vi "Autonomous Independent.vi"   [LabVIEW 2017]
doc: "This VI is called when autonomous begins, and will automatically be terminated when autonomous ends. You can carry out timed or sensor driven robot movement independently without needing to return to the caller."
uses:
  <vilib>/Rock Robotics/Network Tables/NT Read String.vi
  <vilib>/Rock Robotics/WPI/Utilities/WPI_GetSetVariantRefNum.vi
  <vilib>/Rock Robotics/Network Tables/NT Read Number.vi
  Robot Global Data.vi
panel:
  # "Be sure to right-click and choose Data Operations>>Make Current Value default if you want to save the array values with the VI"
types:
  T1 = typedef "WPI_RobotDriveDevRef.ctl" = cluster{"DevStatus":errorcluster, "Motors[]":T2[], "Square Inputs":bool, "Max Output":dbl}
  T2 = typedef "WPI_MotorControlDeviceRef.ctl" = cluster{"DeviceStatus":errorcluster, "Type":T3, "PWM":cluster{"PWM Channel":T4, "DeadBand":T5}, "CAN":cluster{"Device Number":u8, "SetOutput VI Ref":variant, "GetOutput VI Ref":variant, "Enable VI Ref":variant, "Disable VI Ref":variant, "Data":variant}, "Invert":bool, "DIO PWM":cluster{"PWM \"Enable\" Channel":T4, "DIOChannel":T6, "PWM Rate":dbl}}
  T3 = typedef "WPI_MotorControlType.ctl" = enum16{"PWM", "CAN", "DIO PWM"}
  T4 = typedef "FPGA_DIOPWMChannel.ctl" = enum8{"PWM 0", "PWM 1", "PWM 2", "PWM 3", "PWM 4", "PWM 5", "PWM 6", "PWM 7", "PWM 8", "PWM 9", "PWM MXP 0", "PWM MXP 1", "PWM MXP 2", "PWM MXP 3", "PWM MXP 4", "PWM MXP 5", "PWM MXP 6", "PWM MXP 7", "PWM MXP 8", "PWM MXP 9", "Invalid"}
  T5 = typedef "WPI_PWMDeadband.ctl" = cluster{"Name":string, "maxPositivePwm":i32, "minPositivePwm":i32, "centerPwm":i32, "maxNegativePwm":i32, "minNegativePwm":i32, "angularRange":u16}
  T6 = typedef "FPGA_DIOChannel.ctl" = enum8{"DIO 0", "DIO 1", "DIO 2", "DIO 3", "DIO 4", "DIO 5", "DIO 6", "DIO 7", "DIO 8", "DIO 9", "DIO MXP 0", "DIO MXP 1", "DIO MXP 2", "DIO MXP 3", "DIO MXP 4", "DIO MXP 5", "DIO MXP 6", "DIO MXP 7", "DIO MXP 8", "DIO MXP 9", "DIO MXP 10", "DIO MXP 11", "DIO MXP 12", "DIO MXP 13", "DIO MXP 14", "DIO MXP 15", "SPI Port CS1", "SPI Port CS2", "SPI Port CS3", "SPI Port MISO", "SPI Port MOSI", "Invalid"}
  T7 = typedef "WPI_DigitalInputDevRef.ctl" = cluster{"DevStatus":errorcluster, "DIO Channel":T6}
  T8 = typedef "WPI_GyroDevRef.ctl" = cluster{"DevStatus":errorcluster, "Analog Channel":T9, "Gain (VoltsPerDegree/Second)":dbl, "Gyro Type":enum16{"Analog", "XRS450"}, "Handle":i32, "SPI Bus":T10, "Device Found":bool, "Sample Rate":dbl, "Calibrate On Open":bool, "Offset":dbl}
  T9 = typedef "FPGA_AIChannel.ctl" = enum8{"AI 0", "AI 1", "AI 2", "AI 3", "AI MXP 0", "AI MXP 1", "AI MXP 2", "AI MXP 3", "Invalid"}
  T10 = typedef "spi_bus.ctl" = enum16{"SPI On-Board, CS0", "SPI On-Board, CS1", "SPI On-Board, CS2", "SPI On-Board, CS3", "SPI MXP", "Invalid"}
  T11 = typedef "WPI_EncoderDevRef.ctl" = cluster{"DevStatus":errorcluster, "EncoderIndex":T12, "CounterIndex":T13, "DistancePerCount":dbl, "Decoding Type":T14}
  T12 = typedef "FPGA_EncoderIdx.ctl" = enum8{"Enc 0", "Enc 1", "Enc 2", "Enc 3", "Enc 4", "Enc 5", "Enc 6", "Enc 7", "Invalid"}
  T13 = typedef "FPGA_CounterCtrSystemIndex.ctl" = enum8{"Ctr 0", "Ctr 1", "Ctr 2", "Ctr 3", "Ctr 4", "Ctr 5", "Ctr 6", "Ctr 7", "Invalid"}
  T14 = typedef "WPI_EncoderType.ctl" = enum16{"1x", "2x", "4x"}
  T15 = cluster{"Axes[0]":dbl, "Axes[1]":dbl, "Axes[2]":dbl, "Axes[3]":dbl, "Axes[4]":dbl, "Axes[5]":dbl, "Axes[6]":dbl, "Axes[7]":dbl, "Axes[8]":dbl}
  T16 = cluster{"CHECKSUM":u16, "SIGNATURE NUMBER":u16, "X CENTER":u16, "Y CENTER":u16, "TRAGET WIDTH":u16, "TARGET HEIGHT":u16, "X_LOCK":bool, "Y_LOCK":bool}
diagram:
  (unwired) "This function is run in parallel when the autonomous period begins. It will be terminated automatically when the period ends.\n\nNote that all Driver Station inputs are automatically latched and will not change once auto begins."
  # "This tells you the autonomous selected\nfrom the dashboard"
  # "Every 20ms, report that we are running autonomous\ncode. Loop will abort the same time as the VI."
  # "Use time and/or sensors to control how the robot drives."
  # "This tells you the driver position\nand alliance color"
  n1 = while {
    tunnel: [w29] -> w9
    tunnel: [w30] -> w6
    i -> [w25]
    stop <- w20 stop-if-true
    n2 = call <vilib>:"WPI_DriverStationGame Specific Data.vi"() -> ("Game Specific Data"=w35:string)  [unwired: 11 in]
    n3 = call <vilib>:"WPI_DriverStationGame Specific Data.vi"() -> ("Game Specific Data"=w33:string)  [unwired: 11 in]
    n4 = Wait (ms)(milliseconds to wait=u32 10) -> ()  [unwired: 1 out]
    n5 = String Subset(string=w35, length (rest)=1 ("length (rest)")) -> (substring=w29:string)  [unwired: 1 in]
    n6 = String Subset(string=w33, offset (0)=1, length (rest)=1 ("length (rest)")) -> (substring=w30:string)
    n7 = String Length(string=w29) -> (length=w27:i32)
    n8 = String Length(string=w30) -> (length=w28:i32)
    n9 = Greater Than 0?(x=w27) -> (x > 0?=w23:bool)
    n10 = Greater Than 0?(x=w28) -> (x > 0?=w22:bool)
    n11 = Greater Or Equal?(x=w25, y=500) -> (x >= y?=w21:bool)
    n12 = Compound Arithmetic op=OR(w23, w22, w21) -> (w20:bool)
  }
  n13 = call <vilib>:"WPI_DriverStationGet Alliance Info.vi"() -> ()  [unwired: 12 out]
  n14 = while {
    stop <- FALSE stop-if-true
    n15 = call <vilib>:"WPI_DriverStationReport Robot Code State.vi"("Autonomous"=TRUE) -> ()  [unwired: 10 in, 1 out]
    n16 = Wait (ms)(milliseconds to wait=u32 20) -> ()  [unwired: 1 out]
  }
  n17 = global write "Robot Global Data.vi" "Current State"(TRUE ("Current State")) -> ()
  n18 = call <vilib>:"WPI_RobotDriveRefNum Registry Get.vi"("refnum name"="Left and Right Motors") -> ("RobotDriveDevRef"=w12:T1)  [unwired: 9 in, 1 out]
  n19 = call-poly <vilib>:"NT Read Value.vi"("Name"="DB/Slider 0" ("refnum name")) -> ("Numeric"=w7:dbl)  [unwired: 9 in, 1 out]
  n20 = call-poly <vilib>:"NT Read Value.vi"("Name"="DB/Slider 1" ("refnum name")) -> ("Numeric"=w4:dbl)  [unwired: 9 in, 1 out]
  n21 = call-poly <vilib>:"NT Read Value.vi"("Name"="Auto Selector") -> ("String"=w18:string)  [unwired: 9 in, 1 out]
  n22 = call <vilib>:"WPI_DigitalInputRefNum Registry Get.vi"("refnum name"="Infrared") -> ("DigitalInputDevRef"=w1:T7)  [unwired: 9 in, 1 out]
  n23 = call <vilib>:"WPI_GyroRefNum Registry Get.vi"("refnum name"="Gyro") -> ("GyroDevRef"=w10:T8)  [unwired: 9 in, 1 out]
  n24 = call <vilib>:"WPI_EncoderRefNum Registry Get.vi"("refnum name"="Left") -> ("EncoderDevRef"=w15:T11)  [unwired: 9 in, 1 out]
  n25 = call <vilib>:"WPI_EncoderRefNum Registry Get.vi"("refnum name"="Right") -> ("EncoderDevRef"=w14:T11)  [unwired: 9 in, 1 out]
  n26 = case shown="\"Right Scale V2\"" w18 {
    tunnel: w15 -> [w47 w86 w449 w1297 w1563 w1948 w2679 w3428 w4238 w4503 w4890 w5156 w5885 w6662 w7471 w7729 w7754 w7788 w7814]
    tunnel: w14 -> [w46 w87 w450 w1296 w1562 w1949 w2680 w3427 w4237 w4504 w4889 w5155 w5884 w6661 w7472 w7728 w7753 w7789 w7813]
    tunnel: w12 -> [w45 w88 w452 w1299 w1564 w1946 w2677 w3430 w4236 w4502 w4892 w5158 w5887 w6664 w7473 w7730 w7756 w7786 w7811]
    tunnel: w10 -> [w41 w85 w451 w1298 w1565 w1947 w2678 w3429 w4239 w4501 w4891 w5157 w5886 w6663 w7470 w7731 w7755 w7787 w7812]
    tunnel: w9 -> [_ w83 w453 w1293 w1559 w1951 w2675 w3424 w4235 w4499 w4886 w5153 w5890 w6658 w7469 _ _ _ _]
    tunnel: w7 -> [w39 w78 w448 w1295 w1561 w1945 w2676 w3426 w4234 w4505 w4888 w5159 w5888 w6660 w7464 w7725 w7750 w7790 w7816]
    tunnel: w6 -> [_ _ _ w1294 w1560 w1950 w2674 w3425 _ w4500 w4887 w5154 w5889 w6659 _ _ _ _ _]
    tunnel: w4 -> [_ _ _ _ _ _ _ _ _ _ _ _ _ _ _ _ w7749 _ w7810]
    tunnel: w1 -> [_ _ _ _ _ _ _ w3423 _ _ _ _ _ w6657 _ _ _ _ w7815]
    frame "Autoline", Default {
      n27 = flat-sequence {
        tunnel: w47 -> [w63]
        tunnel: w46 -> [w62]
        tunnel: w45 -> [w61]
        tunnel: [w60] -> w44
        tunnel: [w59] -> w43
        tunnel: [w58] -> w42
        tunnel: w41 -> [w57]
        tunnel: [w56] -> w40
        tunnel: w39 -> [w53]
        tunnel: w40 -> [w66]
        tunnel: w42 -> [w65]
        tunnel: w43 -> [w64]
        tunnel: w44 -> [w67]
        frame #0 {
          n28 = Multiply(x=w53, y=1000.0) -> (x*y=w50:dbl)
          n29 = Wait (ms)(milliseconds to wait=10) -> ()  [unwired: 1 out]
          n30 = call <vilib>:"WPI_EncoderReset.vi"("EncoderDevRef"=w62) -> ("EncoderDevRef"=w58:T11)  [unwired: 9 in, 1 out]
          n31 = Equal?(x=w50, y=0.0) -> (x = y?=w51:bool)
          n32 = Greater?(x=w50, y=11000.0) -> (0:w52:bool)
          n33 = call <vilib>:"WPI_RobotDriveTankDrive.vi"("RobotDriveDevRef"=w61) -> ("RobotDriveDevRef"=w60:T1)  [unwired: 8 in, 2 out]
          n34 = Or(x=w52, y=w51) -> ()  [unwired: 1 out]
          n35 = call <vilib>:"WPI_GyroReset.vi"("GyroDevRef"=w57) -> ("GyroDevRef"=w56:T8)  [unwired: 9 in, 1 out]
          n36 = call <vilib>:"WPI_EncoderReset.vi"("EncoderDevRef"=w63) -> ("EncoderDevRef"=w59:T11)  [unwired: 9 in, 1 out]
        }
        frame #1 {
          n37 = flat-sequence {
            tunnel: w67 -> [w73]
            tunnel: w66 -> [w72]
            tunnel: w65 -> [w70]
            tunnel: [w71] -> w68
            tunnel: w64 -> [w69]
            tunnel: w68 -> [w76]
            frame #0 {
              n38 = call "PID Distance.vi"("Distance"=90.0, "Angle"=0.0, "RightEncoder"=w69, "LeftEncoder"=w70, "GyroDevRef"=w72, "RobotDriveDevRef"=w73) -> ("RobotDriveDevRef 2"=w71:T1)  [unwired: 2 in, 3 out]
            }
            frame #1 {
              w77 = 0.0
              n39 = call <vilib>:"WPI_RobotDriveTankDrive.vi"("Right axis value"=w77, "Left axis value"=w77, "RobotDriveDevRef"=w76) -> ()  [unwired: 6 in, 3 out]
            }
          }
        }
      }
    }
    frame "Center Switch" {
      n40 = flat-sequence {
        tunnel: [w110] -> w84
        tunnel: [w109] -> w82
        tunnel: [w108] -> w81
        tunnel: [w107] -> w80
        tunnel: [w106] -> w79
        tunnel: w78 -> [w104]
        tunnel: w83 -> [w110]
        tunnel: w85 -> [w111]
        tunnel: w86 -> [w112]
        tunnel: w87 -> [w113]
        tunnel: w88 -> [w114]
        tunnel: w84 -> [w120]
        tunnel: w82 -> [w119]
        tunnel: w81 -> [w118]
        tunnel: w80 -> [w117]
        tunnel: w79 -> [w116]
        frame #0 {
          w115 = 0.0 ("Left axis value")
          # "Section 1:\nCode initialization"
          n41 = global read "Robot Global Data.vi" "Axes"() -> (w95:dbl[])
          n42 = call <vilib>:"WPI_RobotDriveTankDrive.vi"("Right axis value"=w115, "Left axis value"=w115, "RobotDriveDevRef"=w114) -> ("RobotDriveDevRef"=w109:T1)  [unwired: 6 in, 2 out]
          n43 = global write "Robot Global Data.vi" "Lift_Position"(0.0) -> ()
          n44 = Multiply(x=w104, y=1000.0) -> (x*y=w99:dbl)
          n45 = global write "Robot Global Data.vi" "Raise_Mast"(FALSE ("Current State")) -> ()
          n46 = global write "Robot Global Data.vi" "Current State"(TRUE ("Current State")) -> ()
          n47 = global write "Robot Global Data.vi" "Raise_Mast"(FALSE ("Current State")) -> ()
          n48 = Array To Cluster(array=w95) -> (cluster=w94:T15)
          n49 = Bundle By Name(cluster=w94, "Axes[1]"=-1.0) -> (w93:T15)
          n50 = Greater?(x=w99, y=11000.0) -> (0:w101:bool)
          n51 = Equal?(x=w99, y=0.0) -> (x = y?=w102:bool)
          n52 = Or(x=w101, y=w102) -> ()  [unwired: 1 out]
          n53 = Cluster To Array(cluster=w93) -> (array=w92:dbl[])
          n54 = call <vilib>:"WPI_GyroReset.vi"("GyroDevRef"=w111) -> ("GyroDevRef"=w108:T8)  [unwired: 9 in, 1 out]
          n55 = call <vilib>:"WPI_EncoderReset.vi"("EncoderDevRef"=w112) -> ("EncoderDevRef"=w106:T11)  [unwired: 9 in, 1 out]
          n56 = global write "Robot Global Data.vi" "Axes"(w92) -> ()
          n57 = call <vilib>:"WPI_EncoderReset.vi"("EncoderDevRef"=w113) -> ("EncoderDevRef"=w107:T11)  [unwired: 9 in, 1 out]
          n58 = Wait (ms)(milliseconds to wait=0) -> ()  [unwired: 1 out]
        }
        frame #1 {
          n59 = case shown="\"L\"" w120 {
            tunnel: w119 -> [w140 w281 w302]
            tunnel: w118 -> [w141 w280 w303]
            tunnel: w117 -> [w143 w278 w304]
            tunnel: w116 -> [w142 w279 w305]
            frame "R" {
              n60 = flat-sequence {
                tunnel: [w168] -> w164
                tunnel: [w167] -> w163
                tunnel: [w166] -> w162
                tunnel: [w165] -> w161
                tunnel: w143 -> [w169]
                tunnel: w142 -> [w170]
                tunnel: w141 -> [w172]
                tunnel: w140 -> [w171]
                tunnel: [w180] -> w160
                tunnel: w164 -> [w179]
                tunnel: [w178] -> w159
                tunnel: w163 -> [w178]
                tunnel: [w177] -> w158
                tunnel: w162 -> [w177]
                tunnel: [w176] -> w157
                tunnel: w161 -> [w176]
                tunnel: [w183] -> w139
                tunnel: [w184] -> w137
                tunnel: w160 -> [w185]
                tunnel: w159 -> [w186]
                tunnel: [w190] -> w135
                tunnel: w158 -> [w190]
                tunnel: [w189] -> w133
                tunnel: w157 -> [w189]
                tunnel: w139 -> [w199]
                tunnel: [w199] -> w138
                tunnel: w137 -> [w198]
                tunnel: [w193] -> w136
                tunnel: w135 -> [w197]
                tunnel: [w194] -> w134
                tunnel: w133 -> [w196]
                tunnel: [w195] -> w132
                tunnel: w138 -> [w207]
                tunnel: w136 -> [w206]
                tunnel: w134 -> [w204]
                tunnel: w132 -> [w205]
                tunnel: [w202] -> w156
                tunnel: [w203] -> w155
                tunnel: [w201] -> w154
                tunnel: [w200] -> w153
                tunnel: [w211] -> w152
                tunnel: [w212] -> w151
                tunnel: w156 -> [w220]
                tunnel: w155 -> [w219]
                tunnel: [w223] -> w150
                tunnel: w154 -> [w223]
                tunnel: [w222] -> w149
                tunnel: w153 -> [w222]
                tunnel: [w235] -> w148
                tunnel: [w234] -> w147
                tunnel: [w233] -> w146
                tunnel: w152 -> [w233]
                tunnel: [w232] -> w145
                tunnel: w151 -> [w232]
                tunnel: w150 -> [w225]
                tunnel: w149 -> [w224]
                tunnel: w148 -> [w240]
                tunnel: w147 -> [w239]
                tunnel: w146 -> [w242]
                tunnel: w145 -> [w241]
                tunnel: [w243] -> w144
                tunnel: [w238] -> w127
                tunnel: [w237] -> w124
                tunnel: [w236] -> w121
                tunnel: w144 -> [w257]
                tunnel: [w249] -> w130
                tunnel: [w248] -> w128
                tunnel: w127 -> [w248]
                tunnel: [w247] -> w125
                tunnel: w124 -> [w247]
                tunnel: [w246] -> w122
                tunnel: w121 -> [w246]
                tunnel: [w262] -> w131
                tunnel: w130 -> [w262]
                tunnel: [w261] -> w129
                tunnel: w128 -> [w261]
                tunnel: [w260] -> w126
                tunnel: w125 -> [w260]
                tunnel: [w259] -> w123
                tunnel: w122 -> [w259]
                tunnel: w123 -> [w268]
                tunnel: w126 -> [w267]
                tunnel: w129 -> [w266]
                tunnel: w131 -> [w265]
                frame #0 {
                  n61 = call "PID Distance.vi"("Distance"=20.0, "Angle"=0.0, "RightEncoder"=w169, "LeftEncoder"=w170, "GyroDevRef"=w172, "RobotDriveDevRef"=w171) -> ("RightEncoder 2"=w165:T11, "LeftEncoder 2"=w166:T11, "GyroDevRef 2"=w167:T8, "RobotDriveDevRef 2"=w168:T1)  [unwired: 2 in]
                }
                frame #1 {
                  w181 = 0.0 ("Left axis value")
                  n62 = global write "Robot Global Data.vi" "Raise_Mast"(TRUE ("Current State")) -> ()
                  n63 = Wait (ms)(milliseconds to wait=u32 100) -> ()  [unwired: 1 out]
                  n64 = call <vilib>:"WPI_RobotDriveTankDrive.vi"("Right axis value"=w181, "Left axis value"=w181, "RobotDriveDevRef"=w179) -> ("RobotDriveDevRef"=w180:T1)  [unwired: 6 in, 2 out]
                }
                frame #2 {
                  n65 = call "PID turning.vi"("Angle"=45.0, "GyroDevRef"=w186, "RobotDriveDevRef"=w185) -> ("GyroDevRef 2"=w183:T8, "RobotDriveDevRef 2"=w184:T1)  [unwired: 7 in]
                  n66 = global write "Robot Global Data.vi" "Raise_Mast"(TRUE ("Current State")) -> ()
                }
                frame #3 {
                  w192 = 0.0 ("Left axis value")
                  n67 = call <vilib>:"WPI_EncoderReset.vi"("EncoderDevRef"=w197) -> ("EncoderDevRef"=w194:T11)  [unwired: 9 in, 1 out]
                  n68 = call <vilib>:"WPI_EncoderReset.vi"("EncoderDevRef"=w196) -> ("EncoderDevRef"=w195:T11)  [unwired: 9 in, 1 out]
                  n69 = Wait (ms)(milliseconds to wait=u32 10) -> ()  [unwired: 1 out]
                  n70 = call <vilib>:"WPI_RobotDriveTankDrive.vi"("Right axis value"=w192, "Left axis value"=w192, "RobotDriveDevRef"=w198) -> ("RobotDriveDevRef"=w193:T1)  [unwired: 6 in, 2 out]
                }
                frame #4 {
                  n71 = call "PID Distance.vi"("Distance"=60.0, "Angle"=45.0, "RightEncoder"=w205, "LeftEncoder"=w204, "GyroDevRef"=w207, "RobotDriveDevRef"=w206) -> ("RightEncoder 2"=w200:T11, "LeftEncoder 2"=w201:T11, "GyroDevRef 2"=w203:T8, "RobotDriveDevRef 2"=w202:T1)  [unwired: 2 in]
                  n72 = global write "Robot Global Data.vi" "Raise_Mast"(TRUE ("Current State")) -> ()
                }
                frame #5 {
                  n73 = global read "Robot Global Data.vi" "Axes"() -> (w217:dbl[])
                  n74 = global write "Robot Global Data.vi" "Raise_Mast"(TRUE ("Current State")) -> ()
                  n75 = Array To Cluster(array=w217) -> (cluster=w218:T15)
                  n76 = Bundle By Name(cluster=w218, "Axes[1]"=-1.0) -> (w215:T15)
                  n77 = Cluster To Array(cluster=w215) -> (array=w216:dbl[])
                  n78 = call "PID turning.vi"("Angle"=0.0, "GyroDevRef"=w219, "RobotDriveDevRef"=w220) -> ("GyroDevRef 2"=w211:T8, "RobotDriveDevRef 2"=w212:T1)  [unwired: 7 in]
                  n79 = global write "Robot Global Data.vi" "Axes"(w216) -> ()
                }
                frame #6 {
                  n80 = global read "Robot Global Data.vi" "Axes"() -> (w227:dbl[])
                  n81 = global write "Robot Global Data.vi" "Lift_Position"(2.0) -> ()
                  n82 = Array To Cluster(array=w227) -> (cluster=w226:T15)
                  n83 = Bundle By Name(cluster=w226, "Axes[1]"=-1.0) -> (w229:T15)
                  n84 = Cluster To Array(cluster=w229) -> (array=w228:dbl[])
                  n85 = call <vilib>:"WPI_EncoderReset.vi"("EncoderDevRef"=w224) -> ("EncoderDevRef"=w234:T11)  [unwired: 9 in, 1 out]
                  n86 = global write "Robot Global Data.vi" "Axes"(w228) -> ()
                  n87 = call <vilib>:"WPI_EncoderReset.vi"("EncoderDevRef"=w225) -> ("EncoderDevRef"=w235:T11)  [unwired: 9 in, 1 out]
                }
                frame #7 {
                  n88 = call "PID Distance.vi"("Distance"=50.0, "Angle"=0.0, "RightEncoder"=w239, "LeftEncoder"=w240, "GyroDevRef"=w242, "RobotDriveDevRef"=w241) -> ("RightEncoder 2"=w236:T11, "LeftEncoder 2"=w237:T11, "GyroDevRef 2"=w238:T8, "RobotDriveDevRef 2"=w243:T1)  [unwired: 2 in]
                }
                frame #8 {
                  w258 = 0.0 ("Left axis value")
                  n89 = global read "Robot Global Data.vi" "Axes"() -> (w254:dbl[])
                  n90 = global write "Robot Global Data.vi" "Lift_Position"(2.0) -> ()
                  n91 = Wait (ms)(milliseconds to wait=u32 500) -> ()  [unwired: 1 out]
                  n92 = Array To Cluster(array=w254) -> (cluster=w253:T15)
                  n93 = Bundle By Name(cluster=w253, "Axes[1]"=1.0) -> (w251:T15)
                  n94 = Cluster To Array(cluster=w251) -> (array=w250:dbl[])
                  n95 = call <vilib>:"WPI_RobotDriveTankDrive.vi"("Right axis value"=w258, "Left axis value"=w258, "RobotDriveDevRef"=w257) -> ("RobotDriveDevRef"=w249:T1)  [unwired: 6 in, 2 out]
                  n96 = global write "Robot Global Data.vi" "Axes"(w250) -> ()
                }
                frame #9 {
                  n97 = global write "Robot Global Data.vi" "Current State"(FALSE ("Current State")) -> ()
                  n98 = Wait (ms)(milliseconds to wait=u32 500) -> ()  [unwired: 1 out]
                }
                frame #10 {
                  n99 = global read "Robot Global Data.vi" "Axes"() -> (w276:dbl[])
                  n100 = call "PID Distance.vi"("Distance"=20.0, "Angle"=0.0, "RightEncoder"=w268, "LeftEncoder"=w267, "GyroDevRef"=w266, "RobotDriveDevRef"=w265) -> ()  [unwired: 2 in, 4 out]
                  n101 = global write "Robot Global Data.vi" "Lift_Position"(0.0) -> ()
                  n102 = Array To Cluster(array=w276) -> (cluster=w275:T15)
                  n103 = Bundle By Name(cluster=w275, "Axes[1]"=-1.0) -> (w273:T15)
                  n104 = Cluster To Array(cluster=w273) -> (array=w272:dbl[])
                  n105 = global write "Robot Global Data.vi" "Axes"(w272) -> ()
                }
              }
            }
            frame Default {
              n106 = flat-sequence {
                tunnel: w281 -> [w286]
                tunnel: w280 -> [w285]
                tunnel: w279 -> [w283]
                tunnel: w278 -> [w282]
                tunnel: [w284] -> w277
                tunnel: w277 -> [w289]
                frame #0 {
                  n107 = call "PID Distance.vi"("Distance"=90.0, "Angle"=0.0, "RightEncoder"=w282, "LeftEncoder"=w283, "GyroDevRef"=w285, "RobotDriveDevRef"=w286) -> ("RobotDriveDevRef 2"=w284:T1)  [unwired: 2 in, 3 out]
                }
                frame #1 {
                  w290 = 0.0
                  n108 = call <vilib>:"WPI_RobotDriveTankDrive.vi"("Right axis value"=w290, "Left axis value"=w290, "RobotDriveDevRef"=w289) -> ()  [unwired: 6 in, 3 out]
                }
              }
            }
            frame "L" {
              n109 = flat-sequence {
                tunnel: [w338] -> w334
                tunnel: [w337] -> w333
                tunnel: [w336] -> w332
                tunnel: [w335] -> w331
                tunnel: w304 -> [w339]
                tunnel: w305 -> [w340]
                tunnel: w303 -> [w342]
                tunnel: w302 -> [w341]
                tunnel: [w350] -> w330
                tunnel: w334 -> [w349]
                tunnel: [w348] -> w329
                tunnel: w333 -> [w348]
                tunnel: [w347] -> w328
                tunnel: w332 -> [w347]
                tunnel: [w346] -> w327
                tunnel: w331 -> [w346]
                tunnel: [w354] -> w326
                tunnel: [w355] -> w325
                tunnel: w330 -> [w356]
                tunnel: w329 -> [w353]
                tunnel: [w360] -> w324
                tunnel: w328 -> [w360]
                tunnel: [w359] -> w323
                tunnel: w327 -> [w359]
                tunnel: w326 -> [w369]
                tunnel: [w369] -> w322
                tunnel: w325 -> [w368]
                tunnel: [w363] -> w321
                tunnel: w324 -> [w367]
                tunnel: [w364] -> w320
                tunnel: w323 -> [w366]
                tunnel: [w365] -> w319
                tunnel: w322 -> [w377]
                tunnel: w321 -> [w376]
                tunnel: w320 -> [w374]
                tunnel: w319 -> [w375]
                tunnel: [w372] -> w318
                tunnel: [w373] -> w317
                tunnel: [w371] -> w316
                tunnel: [w370] -> w315
                tunnel: [w381] -> w314
                tunnel: [w382] -> w313
                tunnel: w318 -> [w391]
                tunnel: w317 -> [w390]
                tunnel: [w394] -> w312
                tunnel: w316 -> [w394]
                tunnel: [w393] -> w311
                tunnel: w315 -> [w393]
                tunnel: [w406] -> w310
                tunnel: [w405] -> w309
                tunnel: [w404] -> w308
                tunnel: w314 -> [w404]
                tunnel: [w403] -> w307
                tunnel: w313 -> [w403]
                tunnel: w312 -> [w396]
                tunnel: w311 -> [w395]
                tunnel: w310 -> [w411]
                tunnel: w309 -> [w410]
                tunnel: w308 -> [w413]
                tunnel: w307 -> [w412]
                tunnel: [w414] -> w306
                tunnel: [w409] -> w297
                tunnel: [w408] -> w294
                tunnel: [w407] -> w291
                tunnel: w306 -> [w428]
                tunnel: [w420] -> w300
                tunnel: [w419] -> w298
                tunnel: w297 -> [w419]
                tunnel: [w418] -> w295
                tunnel: w294 -> [w418]
                tunnel: [w417] -> w292
                tunnel: w291 -> [w417]
                tunnel: [w433] -> w301
                tunnel: w300 -> [w433]
                tunnel: [w432] -> w299
                tunnel: w298 -> [w432]
                tunnel: [w431] -> w296
                tunnel: w295 -> [w431]
                tunnel: [w430] -> w293
                tunnel: w292 -> [w430]
                tunnel: w301 -> [w439]
                tunnel: w299 -> [w438]
                tunnel: w296 -> [w437]
                tunnel: w293 -> [w436]
                frame #0 {
                  n110 = call "PID Distance.vi"("Distance"=20.0, "Angle"=0.0, "RightEncoder"=w339, "LeftEncoder"=w340, "GyroDevRef"=w342, "RobotDriveDevRef"=w341) -> ("RightEncoder 2"=w335:T11, "LeftEncoder 2"=w336:T11, "GyroDevRef 2"=w337:T8, "RobotDriveDevRef 2"=w338:T1)  [unwired: 2 in]
                }
                frame #1 {
                  w351 = 0.0 ("Left axis value")
                  n111 = global write "Robot Global Data.vi" "Raise_Mast"(TRUE ("Current State")) -> ()
                  n112 = Wait (ms)(milliseconds to wait=u32 100) -> ()  [unwired: 1 out]
                  n113 = call <vilib>:"WPI_RobotDriveTankDrive.vi"("Right axis value"=w351, "Left axis value"=w351, "RobotDriveDevRef"=w349) -> ("RobotDriveDevRef"=w350:T1)  [unwired: 6 in, 2 out]
                }
                frame #2 {
                  n114 = call "PID turning.vi"("Angle"=-50.0, "GyroDevRef"=w353, "RobotDriveDevRef"=w356) -> ("GyroDevRef 2"=w354:T8, "RobotDriveDevRef 2"=w355:T1)  [unwired: 7 in]
                  n115 = global write "Robot Global Data.vi" "Raise_Mast"(TRUE ("Current State")) -> ()
                }
                frame #3 {
                  w362 = 0.0 ("Left axis value")
                  n116 = call <vilib>:"WPI_EncoderReset.vi"("EncoderDevRef"=w367) -> ("EncoderDevRef"=w364:T11)  [unwired: 9 in, 1 out]
                  n117 = call <vilib>:"WPI_EncoderReset.vi"("EncoderDevRef"=w366) -> ("EncoderDevRef"=w365:T11)  [unwired: 9 in, 1 out]
                  n118 = Wait (ms)(milliseconds to wait=u32 10) -> ()  [unwired: 1 out]
                  n119 = call <vilib>:"WPI_RobotDriveTankDrive.vi"("Right axis value"=w362, "Left axis value"=w362, "RobotDriveDevRef"=w368) -> ("RobotDriveDevRef"=w363:T1)  [unwired: 6 in, 2 out]
                }
                frame #4 {
                  n120 = call "PID Distance.vi"("Distance"=75.0, "Angle"=-50.0, "RightEncoder"=w375, "LeftEncoder"=w374, "GyroDevRef"=w377, "RobotDriveDevRef"=w376) -> ("RightEncoder 2"=w370:T11, "LeftEncoder 2"=w371:T11, "GyroDevRef 2"=w373:T8, "RobotDriveDevRef 2"=w372:T1)  [unwired: 2 in]
                  n121 = global write "Robot Global Data.vi" "Raise_Mast"(TRUE ("Current State")) -> ()
                }
                frame #5 {
                  n122 = global read "Robot Global Data.vi" "Axes"() -> (w388:dbl[])
                  n123 = global write "Robot Global Data.vi" "Lift_Position"(2.0) -> ()
                  n124 = global write "Robot Global Data.vi" "Raise_Mast"(TRUE ("Current State")) -> ()
                  n125 = Array To Cluster(array=w388) -> (cluster=w389:T15)
                  n126 = Bundle By Name(cluster=w389, "Axes[1]"=-1.0) -> (w386:T15)
                  n127 = Cluster To Array(cluster=w386) -> (array=w387:dbl[])
                  n128 = call "PID turning.vi"("Angle"=0.0, "GyroDevRef"=w390, "RobotDriveDevRef"=w391) -> ("GyroDevRef 2"=w381:T8, "RobotDriveDevRef 2"=w382:T1)  [unwired: 7 in]
                  n129 = global write "Robot Global Data.vi" "Axes"(w387) -> ()
                }
                frame #6 {
                  n130 = global read "Robot Global Data.vi" "Axes"() -> (w398:dbl[])
                  n131 = global write "Robot Global Data.vi" "Lift_Position"(2.0) -> ()
                  n132 = Array To Cluster(array=w398) -> (cluster=w397:T15)
                  n133 = Bundle By Name(cluster=w397, "Axes[1]"=-1.0) -> (w400:T15)
                  n134 = Cluster To Array(cluster=w400) -> (array=w399:dbl[])
                  n135 = call <vilib>:"WPI_EncoderReset.vi"("EncoderDevRef"=w395) -> ("EncoderDevRef"=w405:T11)  [unwired: 9 in, 1 out]
                  n136 = global write "Robot Global Data.vi" "Axes"(w399) -> ()
                  n137 = call <vilib>:"WPI_EncoderReset.vi"("EncoderDevRef"=w396) -> ("EncoderDevRef"=w406:T11)  [unwired: 9 in, 1 out]
                }
                frame #7 {
                  n138 = call "PID Distance.vi"("Distance"=50.0, "Angle"=0.0, "RightEncoder"=w410, "LeftEncoder"=w411, "GyroDevRef"=w413, "RobotDriveDevRef"=w412) -> ("RightEncoder 2"=w407:T11, "LeftEncoder 2"=w408:T11, "GyroDevRef 2"=w409:T8, "RobotDriveDevRef 2"=w414:T1)  [unwired: 2 in]
                }
                frame #8 {
                  w429 = 0.0 ("Left axis value")
                  n139 = global read "Robot Global Data.vi" "Axes"() -> (w422:dbl[])
                  n140 = global write "Robot Global Data.vi" "Lift_Position"(2.0) -> ()
                  n141 = Wait (ms)(milliseconds to wait=u32 500) -> ()  [unwired: 1 out]
                  n142 = Array To Cluster(array=w422) -> (cluster=w421:T15)
                  n143 = Bundle By Name(cluster=w421, "Axes[1]"=1.0) -> (w424:T15)
                  n144 = Cluster To Array(cluster=w424) -> (array=w423:dbl[])
                  n145 = call <vilib>:"WPI_RobotDriveTankDrive.vi"("Right axis value"=w429, "Left axis value"=w429, "RobotDriveDevRef"=w428) -> ("RobotDriveDevRef"=w420:T1)  [unwired: 6 in, 2 out]
                  n146 = global write "Robot Global Data.vi" "Axes"(w423) -> ()
                }
                frame #9 {
                  n147 = global write "Robot Global Data.vi" "Current State"(FALSE ("Current State")) -> ()
                  n148 = Wait (ms)(milliseconds to wait=u32 500) -> ()  [unwired: 1 out]
                }
                frame #10 {
                  n149 = global read "Robot Global Data.vi" "Axes"() -> (w441:dbl[])
                  n150 = call "PID Distance.vi"("Distance"=10.0, "Angle"=0.0, "RightEncoder"=w436, "LeftEncoder"=w437, "GyroDevRef"=w438, "RobotDriveDevRef"=w439) -> ()  [unwired: 2 in, 4 out]
                  n151 = global write "Robot Global Data.vi" "Lift_Position"(0.0) -> ()
                  n152 = Array To Cluster(array=w441) -> (cluster=w440:T15)
                  n153 = Bundle By Name(cluster=w440, "Axes[1]"=-1.0) -> (w443:T15)
                  n154 = Cluster To Array(cluster=w443) -> (array=w442:dbl[])
                  n155 = global write "Robot Global Data.vi" "Axes"(w442) -> ()
                }
              }
            }
          }
        }
      }
    }
    frame "Center Switch V" {
      n156 = flat-sequence {
        tunnel: [w480] -> w458
        tunnel: [w479] -> w457
        tunnel: [w478] -> w456
        tunnel: [w477] -> w455
        tunnel: [w476] -> w454
        tunnel: w448 -> [w474]
        tunnel: w453 -> [w480]
        tunnel: w451 -> [w481]
        tunnel: w449 -> [w482]
        tunnel: w450 -> [w483]
        tunnel: w452 -> [w484]
        tunnel: w458 -> [w490]
        tunnel: w457 -> [w489]
        tunnel: w456 -> [w488]
        tunnel: w455 -> [w487]
        tunnel: w454 -> [w486]
        frame #0 {
          w485 = 0.0 ("Left axis value")
          # "Section 1:\nCode initialization"
          n157 = global read "Robot Global Data.vi" "Axes"() -> (w465:dbl[])
          n158 = call <vilib>:"WPI_RobotDriveTankDrive.vi"("Right axis value"=w485, "Left axis value"=w485, "RobotDriveDevRef"=w484) -> ("RobotDriveDevRef"=w479:T1)  [unwired: 6 in, 2 out]
          n159 = global write "Robot Global Data.vi" "Lift_Position"(0.0) -> ()
          n160 = Multiply(x=w474, y=1000.0) -> (x*y=w469:dbl)
          n161 = global write "Robot Global Data.vi" "Raise_Mast"(FALSE ("Current State")) -> ()
          n162 = global write "Robot Global Data.vi" "Current State"(TRUE ("Current State")) -> ()
          n163 = global write "Robot Global Data.vi" "Raise_Mast"(FALSE ("Current State")) -> ()
          n164 = Array To Cluster(array=w465) -> (cluster=w464:T15)
          n165 = Bundle By Name(cluster=w464, "Axes[1]"=-1.0) -> (w463:T15)
          n166 = Greater?(x=w469, y=11000.0) -> (0:w471:bool)
          n167 = Equal?(x=w469, y=0.0) -> (x = y?=w472:bool)
          n168 = Or(x=w471, y=w472) -> ()  [unwired: 1 out]
          n169 = Cluster To Array(cluster=w463) -> (array=w462:dbl[])
          n170 = call <vilib>:"WPI_GyroReset.vi"("GyroDevRef"=w481) -> ("GyroDevRef"=w478:T8)  [unwired: 9 in, 1 out]
          n171 = call <vilib>:"WPI_EncoderReset.vi"("EncoderDevRef"=w482) -> ("EncoderDevRef"=w476:T11)  [unwired: 9 in, 1 out]
          n172 = global write "Robot Global Data.vi" "Axes"(w462) -> ()
          n173 = call <vilib>:"WPI_EncoderReset.vi"("EncoderDevRef"=w483) -> ("EncoderDevRef"=w477:T11)  [unwired: 9 in, 1 out]
          n174 = Wait (ms)(milliseconds to wait=0) -> ()  [unwired: 1 out]
        }
        frame #1 {
          n175 = case shown="\"R\"" w490 {
            tunnel: w489 -> [w578 w889 w902]
            tunnel: w488 -> [w579 w888 w901]
            tunnel: w487 -> [w581 w886 w899]
            tunnel: w486 -> [w580 w887 w900]
            frame "R" {
              n176 = flat-sequence {
                tunnel: [w606] -> w602
                tunnel: [w605] -> w601
                tunnel: [w604] -> w600
                tunnel: [w603] -> w599
                tunnel: w581 -> [w607]
                tunnel: w580 -> [w608]
                tunnel: w579 -> [w610]
                tunnel: w578 -> [w609]
                tunnel: [w618] -> w598
                tunnel: w602 -> [w617]
                tunnel: [w616] -> w597
                tunnel: w601 -> [w616]
                tunnel: [w615] -> w596
                tunnel: w600 -> [w615]
                tunnel: [w614] -> w595
                tunnel: w599 -> [w614]
                tunnel: [w621] -> w577
                tunnel: [w622] -> w575
                tunnel: w598 -> [w623]
                tunnel: w597 -> [w624]
                tunnel: [w628] -> w573
                tunnel: w596 -> [w628]
                tunnel: [w627] -> w571
                tunnel: w595 -> [w627]
                tunnel: w577 -> [w637]
                tunnel: [w637] -> w576
                tunnel: w575 -> [w636]
                tunnel: [w631] -> w574
                tunnel: w573 -> [w635]
                tunnel: [w632] -> w572
                tunnel: w571 -> [w634]
                tunnel: [w633] -> w570
                tunnel: w576 -> [w645]
                tunnel: w574 -> [w644]
                tunnel: w572 -> [w642]
                tunnel: w570 -> [w643]
                tunnel: [w640] -> w594
                tunnel: [w641] -> w593
                tunnel: [w639] -> w592
                tunnel: [w638] -> w591
                tunnel: [w649] -> w590
                tunnel: [w650] -> w589
                tunnel: w594 -> [w658]
                tunnel: w593 -> [w657]
                tunnel: [w661] -> w588
                tunnel: w592 -> [w661]
                tunnel: [w660] -> w587
                tunnel: w591 -> [w660]
                tunnel: [w673] -> w586
                tunnel: [w672] -> w585
                tunnel: [w671] -> w584
                tunnel: w590 -> [w671]
                tunnel: [w670] -> w583
                tunnel: w589 -> [w670]
                tunnel: w588 -> [w663]
                tunnel: w587 -> [w662]
                tunnel: w586 -> [w678]
                tunnel: w585 -> [w677]
                tunnel: w584 -> [w680]
                tunnel: w583 -> [w679]
                tunnel: [w681] -> w582
                tunnel: [w676] -> w565
                tunnel: [w675] -> w562
                tunnel: [w674] -> w559
                tunnel: w582 -> [w695]
                tunnel: [w687] -> w568
                tunnel: [w686] -> w566
                tunnel: w565 -> [w686]
                tunnel: [w685] -> w563
                tunnel: w562 -> [w685]
                tunnel: [w684] -> w560
                tunnel: w559 -> [w684]
                tunnel: [w700] -> w569
                tunnel: w568 -> [w700]
                tunnel: [w699] -> w567
                tunnel: w566 -> [w699]
                tunnel: [w698] -> w564
                tunnel: w563 -> [w698]
                tunnel: [w697] -> w561
                tunnel: w560 -> [w697]
                tunnel: w561 -> [w710]
                tunnel: w564 -> [w709]
                tunnel: w567 -> [w708]
                tunnel: w569 -> [w707]
                tunnel: [w706] -> w558
                tunnel: [w705] -> w557
                tunnel: [w704] -> w555
                tunnel: [w703] -> w553
                tunnel: w558 -> [w724]
                tunnel: w557 -> [w723]
                tunnel: [w722] -> w556
                tunnel: w555 -> [w722]
                tunnel: [w721] -> w554
                tunnel: w553 -> [w721]
                tunnel: [w720] -> w551
                tunnel: [w719] -> w549
                tunnel: w556 -> [w731]
                tunnel: w554 -> [w730]
                tunnel: [w729] -> w552
                tunnel: w551 -> [w729]
                tunnel: [w728] -> w550
                tunnel: w549 -> [w728]
                tunnel: [w727] -> w548
                tunnel: [w726] -> w547
                tunnel: w552 -> [w740]
                tunnel: w550 -> [w739]
                tunnel: w548 -> [w738]
                tunnel: w547 -> [w737]
                tunnel: [w736] -> w546
                tunnel: [w735] -> w545
                tunnel: [w734] -> w540
                tunnel: [w733] -> w537
                tunnel: w546 -> [w748]
                tunnel: w545 -> [w747]
                tunnel: [w746] -> w544
                tunnel: [w745] -> w543
                tunnel: [w744] -> w541
                tunnel: w540 -> [w744]
                tunnel: [w743] -> w538
                tunnel: w537 -> [w743]
                tunnel: w544 -> [w756]
                tunnel: w543 -> [w755]
                tunnel: [w754] -> w542
                tunnel: w541 -> [w754]
                tunnel: [w753] -> w539
                tunnel: w538 -> [w753]
                tunnel: [w752] -> w535
                tunnel: [w751] -> w533
                tunnel: w542 -> [w776]
                tunnel: w539 -> [w775]
                tunnel: [w774] -> w536
                tunnel: w535 -> [w774]
                tunnel: [w773] -> w534
                tunnel: w533 -> [w773]
                tunnel: [w772] -> w532
                tunnel: [w771] -> w531
                tunnel: w536 -> [w784]
                tunnel: w534 -> [w783]
                tunnel: w532 -> [w782]
                tunnel: w531 -> [w781]
                tunnel: [w780] -> w529
                tunnel: [w779] -> w527
                tunnel: [w778] -> w525
                tunnel: [w777] -> w523
                tunnel: [w790] -> w530
                tunnel: w529 -> [w790]
                tunnel: [w789] -> w528
                tunnel: w527 -> [w789]
                tunnel: [w788] -> w526
                tunnel: w525 -> [w788]
                tunnel: [w787] -> w524
                tunnel: w523 -> [w787]
                tunnel: [w798] -> w522
                tunnel: [w794] -> w521
                tunnel: [w793] -> w520
                tunnel: [w797] -> w518
                tunnel: w524 -> [w793]
                tunnel: w526 -> [w794]
                tunnel: w528 -> [w795]
                tunnel: w530 -> [w796]
                tunnel: w522 -> [w806]
                tunnel: w521 -> [w805]
                tunnel: w520 -> [w804]
                tunnel: [w803] -> w519
                tunnel: w518 -> [w803]
                tunnel: [w802] -> w517
                tunnel: [w801] -> w516
                tunnel: [w800] -> w515
                tunnel: w519 -> [w816]
                tunnel: w517 -> [w815]
                tunnel: w516 -> [w814]
                tunnel: w515 -> [w813]
                tunnel: [w812] -> w514
                tunnel: [w811] -> w513
                tunnel: [w810] -> w511
                tunnel: [w809] -> w509
                tunnel: w514 -> [w825]
                tunnel: w513 -> [w824]
                tunnel: [w823] -> w512
                tunnel: w511 -> [w823]
                tunnel: [w822] -> w510
                tunnel: w509 -> [w822]
                tunnel: [w821] -> w507
                tunnel: [w820] -> w505
                tunnel: w512 -> [w838]
                tunnel: w510 -> [w837]
                tunnel: [w836] -> w508
                tunnel: w507 -> [w836]
                tunnel: [w835] -> w506
                tunnel: w505 -> [w835]
                tunnel: [w834] -> w504
                tunnel: [w833] -> w503
                tunnel: w508 -> [w852]
                tunnel: w506 -> [w851]
                tunnel: w504 -> [w850]
                tunnel: w503 -> [w849]
                tunnel: [w848] -> w500
                tunnel: [w847] -> w497
                tunnel: [w846] -> w494
                tunnel: [w845] -> w491
                tunnel: [w858] -> w501
                tunnel: w500 -> [w859]
                tunnel: [w857] -> w498
                tunnel: w497 -> [w857]
                tunnel: [w856] -> w495
                tunnel: w494 -> [w856]
                tunnel: [w855] -> w492
                tunnel: w491 -> [w855]
                tunnel: [w870] -> w502
                tunnel: w501 -> [w870]
                tunnel: [w869] -> w499
                tunnel: w498 -> [w869]
                tunnel: [w868] -> w496
                tunnel: w495 -> [w868]
                tunnel: [w867] -> w493
                tunnel: w492 -> [w867]
                tunnel: w502 -> [w876]
                tunnel: w499 -> [w875]
                tunnel: w496 -> [w874]
                tunnel: w493 -> [w873]
                frame #0 {
                  n177 = call "PID Distance.vi"("Distance"=20.0, "Angle"=0.0, "RightEncoder"=w607, "LeftEncoder"=w608, "GyroDevRef"=w610, "RobotDriveDevRef"=w609) -> ("RightEncoder 2"=w603:T11, "LeftEncoder 2"=w604:T11, "GyroDevRef 2"=w605:T8, "RobotDriveDevRef 2"=w606:T1)  [unwired: 2 in]
                }
                frame #1 {
                  w619 = 0.0 ("Left axis value")
                  n178 = global write "Robot Global Data.vi" "Raise_Mast"(TRUE ("Current State")) -> ()
                  n179 = Wait (ms)(milliseconds to wait=u32 100) -> ()  [unwired: 1 out]
                  n180 = call <vilib>:"WPI_RobotDriveTankDrive.vi"("Right axis value"=w619, "Left axis value"=w619, "RobotDriveDevRef"=w617) -> ("RobotDriveDevRef"=w618:T1)  [unwired: 6 in, 2 out]
                }
                frame #2 {
                  n181 = call "PID turning.vi"("Angle"=45.0, "GyroDevRef"=w624, "RobotDriveDevRef"=w623) -> ("GyroDevRef 2"=w621:T8, "RobotDriveDevRef 2"=w622:T1)  [unwired: 7 in]
                  n182 = global write "Robot Global Data.vi" "Raise_Mast"(TRUE ("Current State")) -> ()
                }
                frame #3 {
                  w630 = 0.0 ("Left axis value")
                  n183 = call <vilib>:"WPI_EncoderReset.vi"("EncoderDevRef"=w635) -> ("EncoderDevRef"=w632:T11)  [unwired: 9 in, 1 out]
                  n184 = call <vilib>:"WPI_EncoderReset.vi"("EncoderDevRef"=w634) -> ("EncoderDevRef"=w633:T11)  [unwired: 9 in, 1 out]
                  n185 = Wait (ms)(milliseconds to wait=u32 10) -> ()  [unwired: 1 out]
                  n186 = call <vilib>:"WPI_RobotDriveTankDrive.vi"("Right axis value"=w630, "Left axis value"=w630, "RobotDriveDevRef"=w636) -> ("RobotDriveDevRef"=w631:T1)  [unwired: 6 in, 2 out]
                }
                frame #4 {
                  n187 = call "PID Distance.vi"("Distance"=60.0, "Angle"=45.0, "RightEncoder"=w643, "LeftEncoder"=w642, "GyroDevRef"=w645, "RobotDriveDevRef"=w644) -> ("RightEncoder 2"=w638:T11, "LeftEncoder 2"=w639:T11, "GyroDevRef 2"=w641:T8, "RobotDriveDevRef 2"=w640:T1)  [unwired: 2 in]
                  n188 = global write "Robot Global Data.vi" "Raise_Mast"(TRUE ("Current State")) -> ()
                }
                frame #5 {
                  n189 = global read "Robot Global Data.vi" "Axes"() -> (w655:dbl[])
                  n190 = global write "Robot Global Data.vi" "Raise_Mast"(TRUE ("Current State")) -> ()
                  n191 = Array To Cluster(array=w655) -> (cluster=w656:T15)
                  n192 = Bundle By Name(cluster=w656, "Axes[1]"=-1.0) -> (w653:T15)
                  n193 = Cluster To Array(cluster=w653) -> (array=w654:dbl[])
                  n194 = call "PID turning.vi"("Angle"=0.0, "GyroDevRef"=w657, "RobotDriveDevRef"=w658) -> ("GyroDevRef 2"=w649:T8, "RobotDriveDevRef 2"=w650:T1)  [unwired: 7 in]
                  n195 = global write "Robot Global Data.vi" "Axes"(w654) -> ()
                }
                frame #6 {
                  n196 = global read "Robot Global Data.vi" "Axes"() -> (w665:dbl[])
                  n197 = global write "Robot Global Data.vi" "Lift_Position"(2.0) -> ()
                  n198 = Array To Cluster(array=w665) -> (cluster=w664:T15)
                  n199 = Bundle By Name(cluster=w664, "Axes[1]"=-1.0) -> (w667:T15)
                  n200 = Cluster To Array(cluster=w667) -> (array=w666:dbl[])
                  n201 = call <vilib>:"WPI_EncoderReset.vi"("EncoderDevRef"=w662) -> ("EncoderDevRef"=w672:T11)  [unwired: 9 in, 1 out]
                  n202 = global write "Robot Global Data.vi" "Axes"(w666) -> ()
                  n203 = call <vilib>:"WPI_EncoderReset.vi"("EncoderDevRef"=w663) -> ("EncoderDevRef"=w673:T11)  [unwired: 9 in, 1 out]
                }
                frame #7 {
                  n204 = call "PID Distance.vi"("Distance"=50.0, "Angle"=0.0, "RightEncoder"=w677, "LeftEncoder"=w678, "GyroDevRef"=w680, "RobotDriveDevRef"=w679) -> ("RightEncoder 2"=w674:T11, "LeftEncoder 2"=w675:T11, "GyroDevRef 2"=w676:T8, "RobotDriveDevRef 2"=w681:T1)  [unwired: 2 in]
                }
                frame #8 {
                  w696 = 0.0 ("Left axis value")
                  n205 = global read "Robot Global Data.vi" "Axes"() -> (w692:dbl[])
                  n206 = global write "Robot Global Data.vi" "Lift_Position"(2.0) -> ()
                  n207 = Wait (ms)(milliseconds to wait=u32 250) -> ()  [unwired: 1 out]
                  n208 = Array To Cluster(array=w692) -> (cluster=w691:T15)
                  n209 = Bundle By Name(cluster=w691, "Axes[1]"=1.0) -> (w689:T15)
                  n210 = Cluster To Array(cluster=w689) -> (array=w688:dbl[])
                  n211 = call <vilib>:"WPI_RobotDriveTankDrive.vi"("Right axis value"=w696, "Left axis value"=w696, "RobotDriveDevRef"=w695) -> ("RobotDriveDevRef"=w687:T1)  [unwired: 6 in, 2 out]
                  n212 = global write "Robot Global Data.vi" "Axes"(w688) -> ()
                }
                frame #9 {
                  n213 = global write "Robot Global Data.vi" "Current State"(FALSE ("Current State")) -> ()
                  n214 = Wait (ms)(milliseconds to wait=u32 500) -> ()  [unwired: 1 out]
                }
                frame #10 {
                  n215 = global read "Robot Global Data.vi" "Axes"() -> (w718:dbl[])
                  n216 = global write "Robot Global Data.vi" "Lift_Position"(1.0) -> ()
                  n217 = Array To Cluster(array=w718) -> (cluster=w717:T15)
                  n218 = Bundle By Name(cluster=w717, "Axes[1]"=0.0) -> (w715:T15)
                  n219 = Cluster To Array(cluster=w715) -> (array=w714:dbl[])
                  n220 = call "PID Distance.vi"("Distance"=0.0, "Angle"=0.0, "RightEncoder"=w710, "LeftEncoder"=w709, "GyroDevRef"=w708, "RobotDriveDevRef"=w707) -> ("RightEncoder 2"=w703:T11, "LeftEncoder 2"=w704:T11, "GyroDevRef 2"=w705:T8, "RobotDriveDevRef 2"=w706:T1)  [unwired: 2 in]
                  n221 = global write "Robot Global Data.vi" "Axes"(w714) -> ()
                }
                frame #11 {
                  n222 = call "PID turning.vi"("Angle"=45.0, "GyroDevRef"=w723, "RobotDriveDevRef"=w724) -> ("GyroDevRef 2"=w719:T8, "RobotDriveDevRef 2"=w720:T1)  [unwired: 7 in]
                }
                frame #12 {
                  n223 = call <vilib>:"WPI_EncoderReset.vi"("EncoderDevRef"=w731) -> ("EncoderDevRef"=w727:T11)  [unwired: 9 in, 1 out]
                  n224 = call <vilib>:"WPI_EncoderReset.vi"("EncoderDevRef"=w730) -> ("EncoderDevRef"=w726:T11)  [unwired: 9 in, 1 out]
                }
                frame #13 {
                  n225 = global write "Robot Global Data.vi" "Lift_Position"(0.0) -> ()
                  n226 = call "PID Distance.vi"("Distance"=-60.0, "Angle"=45.0, "RightEncoder"=w737, "LeftEncoder"=w738, "GyroDevRef"=w739, "RobotDriveDevRef"=w740) -> ("RightEncoder 2"=w733:T11, "LeftEncoder 2"=w734:T11, "GyroDevRef 2"=w735:T8, "RobotDriveDevRef 2"=w736:T1)  [unwired: 2 in]
                }
                frame #14 {
                  n227 = call "PID turning.vi"("Angle"=0.0, "GyroDevRef"=w747, "RobotDriveDevRef"=w748) -> ("GyroDevRef 2"=w745:T8, "RobotDriveDevRef 2"=w746:T1)  [unwired: 7 in]
                }
                frame #15 {
                  n228 = global read "Robot Global Data.vi" "PIXY Output"() -> (w757:T16)
                  n229 = Unbundle By Name(w757) -> ("SIGNATURE NUMBER"=w759:u16)
                  n230 = global read "Robot Global Data.vi" "Cube Signature"() -> (w750:dbl)
                  n231 = Equal?(x=w759, y=w750) -> (x = y?=w758:bool)
                  n232 = case shown="True" w758 {
                    tunnel: [w766 w769] -> w751
                    tunnel: [w767 w768] -> w752
                    tunnel: w756 -> [w761 w768]
                    tunnel: w755 -> [w760 w769]
                    frame True {
                      n233 = call <vilib>:"WPI_GyroGetAngle.vi"("GyroDevRef"=w760) -> ("Angle"=w765:dbl, "GyroDevRef"=w766:T8)  [unwired: 6 in, 3 out]
                      n234 = In Range and Coerce(upper limit=-1.0, x=w765, lower limit=-5.0) -> (coerced(x)=w764:dbl)  [unwired: 1 out]
                      n235 = global write "Robot Global Data.vi" "Tracked Angle"(w764) -> ()
                      n236 = call "PID vision.vi"("RobotDriveDevRef in"=w761) -> ("RobotDriveDevRef out"=w767:T1)  [unwired: 9 in, 1 out]
                    }
                    frame False {
                      n237 = global write "Robot Global Data.vi" "Tracked Angle"(-2.0) -> ()
                    }
                  }
                }
                frame #16 {
                  n238 = call <vilib>:"WPI_EncoderReset.vi"("EncoderDevRef"=w776) -> ("EncoderDevRef"=w772:T11)  [unwired: 9 in, 1 out]
                  n239 = call <vilib>:"WPI_EncoderReset.vi"("EncoderDevRef"=w775) -> ("EncoderDevRef"=w771:T11)  [unwired: 9 in, 1 out]
                }
                frame #17 {
                  n240 = global read "Robot Global Data.vi" "Tracked Angle"() -> (w785:dbl)
                  n241 = call "PID Distance.vi"("Distance"=52.0, "Angle"=w785, "RightEncoder"=w781, "LeftEncoder"=w782, "GyroDevRef"=w783, "RobotDriveDevRef"=w784) -> ("RightEncoder 2"=w777:T11, "LeftEncoder 2"=w778:T11, "GyroDevRef 2"=w779:T8, "RobotDriveDevRef 2"=w780:T1)  [unwired: 2 in]
                }
                frame #18 {
                  n242 = global write "Robot Global Data.vi" "Current State"(TRUE ("Current State")) -> ()
                  n243 = Wait (ms)(milliseconds to wait=u32 750) -> ()  [unwired: 1 out]
                }
                frame #19 {
                  n244 = call "PID turning.vi"("Angle"=90.0, "GyroDevRef"=w795, "RobotDriveDevRef"=w796) -> ("GyroDevRef 2"=w797:T8, "RobotDriveDevRef 2"=w798:T1)  [unwired: 7 in]
                }
                frame #20 {
                  w807 = 0.0 ("Left axis value")
                  n245 = call <vilib>:"WPI_EncoderReset.vi"("EncoderDevRef"=w805) -> ("EncoderDevRef"=w801:T11)  [unwired: 9 in, 1 out]
                  n246 = call <vilib>:"WPI_RobotDriveTankDrive.vi"("Right axis value"=w807, "Left axis value"=w807, "RobotDriveDevRef"=w806) -> ("RobotDriveDevRef"=w802:T1)  [unwired: 6 in, 2 out]
                  n247 = Wait (ms)(milliseconds to wait=u32 10) -> ()  [unwired: 1 out]
                  n248 = call <vilib>:"WPI_EncoderReset.vi"("EncoderDevRef"=w804) -> ("EncoderDevRef"=w800:T11)  [unwired: 9 in, 1 out]
                }
                frame #21 {
                  n249 = call "PID Distance.vi"("Distance"=50.0, "Angle"=90.0, "RightEncoder"=w813, "LeftEncoder"=w814, "GyroDevRef"=w816, "RobotDriveDevRef"=w815) -> ("RightEncoder 2"=w809:T11, "LeftEncoder 2"=w810:T11, "GyroDevRef 2"=w811:T8, "RobotDriveDevRef 2"=w812:T1)  [unwired: 2 in]
                  n250 = global write "Robot Global Data.vi" "Raise_Mast"(TRUE ("Current State")) -> ()
                }
                frame #22 {
                  n251 = global read "Robot Global Data.vi" "Axes"() -> (w830:dbl[])
                  n252 = global write "Robot Global Data.vi" "Raise_Mast"(TRUE ("Current State")) -> ()
                  n253 = Array To Cluster(array=w830) -> (cluster=w831:T15)
                  n254 = Bundle By Name(cluster=w831, "Axes[1]"=-1.0) -> (w828:T15)
                  n255 = Cluster To Array(cluster=w828) -> (array=w829:dbl[])
                  n256 = call "PID turning.vi"("Angle"=0.0, "GyroDevRef"=w824, "RobotDriveDevRef"=w825) -> ("GyroDevRef 2"=w820:T8, "RobotDriveDevRef 2"=w821:T1)  [unwired: 7 in]
                  n257 = global write "Robot Global Data.vi" "Axes"(w829) -> ()
                }
                frame #23 {
                  n258 = global read "Robot Global Data.vi" "Axes"() -> (w840:dbl[])
                  n259 = global write "Robot Global Data.vi" "Lift_Position"(2.0) -> ()
                  n260 = Array To Cluster(array=w840) -> (cluster=w839:T15)
                  n261 = Bundle By Name(cluster=w839, "Axes[1]"=-1.0) -> (w842:T15)
                  n262 = Cluster To Array(cluster=w842) -> (array=w841:dbl[])
                  n263 = call <vilib>:"WPI_EncoderReset.vi"("EncoderDevRef"=w837) -> ("EncoderDevRef"=w833:T11)  [unwired: 9 in, 1 out]
                  n264 = global write "Robot Global Data.vi" "Axes"(w841) -> ()
                  n265 = call <vilib>:"WPI_EncoderReset.vi"("EncoderDevRef"=w838) -> ("EncoderDevRef"=w834:T11)  [unwired: 9 in, 1 out]
                }
                frame #24 {
                  n266 = call "PID Distance.vi"("Distance"=40.0, "Angle"=0.0, "RightEncoder"=w849, "LeftEncoder"=w850, "GyroDevRef"=w851, "RobotDriveDevRef"=w852) -> ("RightEncoder 2"=w845:T11, "LeftEncoder 2"=w846:T11, "GyroDevRef 2"=w847:T8, "RobotDriveDevRef 2"=w848:T1)  [unwired: 2 in]
                }
                frame #25 {
                  w866 = 0.0 ("Left axis value")
                  n267 = global read "Robot Global Data.vi" "Axes"() -> (w864:dbl[])
                  n268 = global write "Robot Global Data.vi" "Lift_Position"(2.0) -> ()
                  n269 = Array To Cluster(array=w864) -> (cluster=w863:T15)
                  n270 = Bundle By Name(cluster=w863, "Axes[1]"=1.0) -> (w861:T15)
                  n271 = Cluster To Array(cluster=w861) -> (array=w860:dbl[])
                  n272 = call <vilib>:"WPI_RobotDriveTankDrive.vi"("Right axis value"=w866, "Left axis value"=w866, "RobotDriveDevRef"=w859) -> ("RobotDriveDevRef"=w858:T1)  [unwired: 6 in, 2 out]
                  n273 = global write "Robot Global Data.vi" "Axes"(w860) -> ()
                }
                frame #26 {
                  n274 = global write "Robot Global Data.vi" "Current State"(FALSE ("Current State")) -> ()
                  n275 = Wait (ms)(milliseconds to wait=u32 500) -> ()  [unwired: 1 out]
                }
                frame #27 {
                  n276 = global read "Robot Global Data.vi" "Axes"() -> (w884:dbl[])
                  n277 = call "PID Distance.vi"("Distance"=0.0, "Angle"=0.0, "RightEncoder"=w873, "LeftEncoder"=w874, "GyroDevRef"=w875, "RobotDriveDevRef"=w876) -> ()  [unwired: 2 in, 4 out]
                  n278 = global write "Robot Global Data.vi" "Lift_Position"(0.0) -> ()
                  n279 = Array To Cluster(array=w884) -> (cluster=w883:T15)
                  n280 = Bundle By Name(cluster=w883, "Axes[1]"=0.0) -> (w878:T15)
                  n281 = Cluster To Array(cluster=w878) -> (array=w877:dbl[])
                  n282 = global write "Robot Global Data.vi" "Axes"(w877) -> ()
                }
              }
            }
            frame Default {
              n283 = flat-sequence {
                tunnel: w889 -> [w894]
                tunnel: w888 -> [w893]
                tunnel: w887 -> [w891]
                tunnel: w886 -> [w890]
                tunnel: [w892] -> w885
                tunnel: w885 -> [w897]
                frame #0 {
                  n284 = call "PID Distance.vi"("Distance"=90.0, "Angle"=0.0, "RightEncoder"=w890, "LeftEncoder"=w891, "GyroDevRef"=w893, "RobotDriveDevRef"=w894) -> ("RobotDriveDevRef 2"=w892:T1)  [unwired: 2 in, 3 out]
                }
                frame #1 {
                  w898 = 0.0
                  n285 = call <vilib>:"WPI_RobotDriveTankDrive.vi"("Right axis value"=w898, "Left axis value"=w898, "RobotDriveDevRef"=w897) -> ()  [unwired: 6 in, 3 out]
                }
              }
            }
            frame "L" {
              n286 = flat-sequence {
                tunnel: [w1014] -> w1010
                tunnel: [w1013] -> w1009
                tunnel: [w1012] -> w1008
                tunnel: [w1011] -> w1007
                tunnel: w899 -> [w1015]
                tunnel: w900 -> [w1016]
                tunnel: w901 -> [w1018]
                tunnel: w902 -> [w1017]
                tunnel: [w1026] -> w1006
                tunnel: w1010 -> [w1025]
                tunnel: [w1024] -> w1005
                tunnel: w1009 -> [w1024]
                tunnel: [w1023] -> w1004
                tunnel: w1008 -> [w1023]
                tunnel: [w1022] -> w1003
                tunnel: w1007 -> [w1022]
                tunnel: [w1029] -> w1002
                tunnel: [w1030] -> w1001
                tunnel: w1006 -> [w1031]
                tunnel: w1005 -> [w1032]
                tunnel: [w1036] -> w1000
                tunnel: w1004 -> [w1036]
                tunnel: [w1035] -> w999
                tunnel: w1003 -> [w1035]
                tunnel: w1002 -> [w1045]
                tunnel: [w1045] -> w998
                tunnel: w1001 -> [w1044]
                tunnel: [w1039] -> w997
                tunnel: w1000 -> [w1043]
                tunnel: [w1040] -> w996
                tunnel: w999 -> [w1042]
                tunnel: [w1041] -> w995
                tunnel: w998 -> [w1053]
                tunnel: w997 -> [w1052]
                tunnel: w996 -> [w1050]
                tunnel: w995 -> [w1051]
                tunnel: [w1048] -> w994
                tunnel: [w1049] -> w993
                tunnel: [w1047] -> w992
                tunnel: [w1046] -> w991
                tunnel: [w1057] -> w990
                tunnel: [w1058] -> w989
                tunnel: w994 -> [w1066]
                tunnel: w993 -> [w1065]
                tunnel: [w1069] -> w988
                tunnel: w992 -> [w1069]
                tunnel: [w1068] -> w987
                tunnel: w991 -> [w1068]
                tunnel: [w1081] -> w986
                tunnel: [w1080] -> w985
                tunnel: [w1079] -> w984
                tunnel: w990 -> [w1079]
                tunnel: [w1078] -> w983
                tunnel: w989 -> [w1078]
                tunnel: w988 -> [w1071]
                tunnel: w987 -> [w1070]
                tunnel: w986 -> [w1086]
                tunnel: w985 -> [w1085]
                tunnel: w984 -> [w1088]
                tunnel: w983 -> [w1087]
                tunnel: [w1089] -> w982
                tunnel: [w1084] -> w981
                tunnel: [w1083] -> w980
                tunnel: [w1082] -> w979
                tunnel: w982 -> [w1103]
                tunnel: [w1095] -> w978
                tunnel: [w1094] -> w977
                tunnel: w981 -> [w1094]
                tunnel: [w1093] -> w976
                tunnel: w980 -> [w1093]
                tunnel: [w1092] -> w975
                tunnel: w979 -> [w1092]
                tunnel: [w1108] -> w971
                tunnel: w978 -> [w1108]
                tunnel: [w1107] -> w972
                tunnel: w977 -> [w1107]
                tunnel: [w1106] -> w973
                tunnel: w976 -> [w1106]
                tunnel: [w1105] -> w974
                tunnel: w975 -> [w1105]
                tunnel: w974 -> [w1118]
                tunnel: w973 -> [w1117]
                tunnel: w972 -> [w1116]
                tunnel: w971 -> [w1115]
                tunnel: [w1114] -> w970
                tunnel: [w1113] -> w969
                tunnel: [w1112] -> w968
                tunnel: [w1111] -> w967
                tunnel: w970 -> [w1132]
                tunnel: w969 -> [w1131]
                tunnel: [w1130] -> w966
                tunnel: w968 -> [w1130]
                tunnel: [w1129] -> w965
                tunnel: w967 -> [w1129]
                tunnel: [w1128] -> w964
                tunnel: [w1127] -> w963
                tunnel: w966 -> [w1139]
                tunnel: w965 -> [w1138]
                tunnel: [w1137] -> w962
                tunnel: w964 -> [w1137]
                tunnel: [w1136] -> w961
                tunnel: w963 -> [w1136]
                tunnel: [w1135] -> w960
                tunnel: [w1134] -> w959
                tunnel: w962 -> [w1148]
                tunnel: w961 -> [w1147]
                tunnel: w960 -> [w1146]
                tunnel: w959 -> [w1145]
                tunnel: [w1144] -> w958
                tunnel: [w1143] -> w957
